vi "Configure Channel.vi"(8 "error in (no error)":errorcluster, 10 "DAQmx Task In":refnum<k21>, 11 "DAQmxThermocoupleChannel in":refnum<class "TCChannel.lvclass">) -> (0 "error out":errorcluster, 2 "DAQmx Task":refnum<k21>)   [LabVIEW 2020, in "VolatusDAQConfig.lvlib" / "TCChannel.lvclass"]
uses:
  TCChannel.lvclass
  VolatusConfig/VolatusConfigElement/VolatusConfigElement.lvclass
  VolatusConfig/Channel/Channel.lvclass
  <vilib>/DAQmx/create/channels.llb/DAQmx Create Channel (AI-Temperature-Thermocouple).vi
  C:/dev/lv20CE/relink/lv-volatus/VolatusDAQConfig/DAQmxChannel/DAQmxChannel.lvclass
  C:/dev/lv20CE/relink/lv-volatus/VolatusConfig/Channel/Channel.lvclass
  C:/dev/lv20CE/relink/lv-volatus/VolatusConfig/VolatusConfigElement/VolatusConfigElement.lvclass
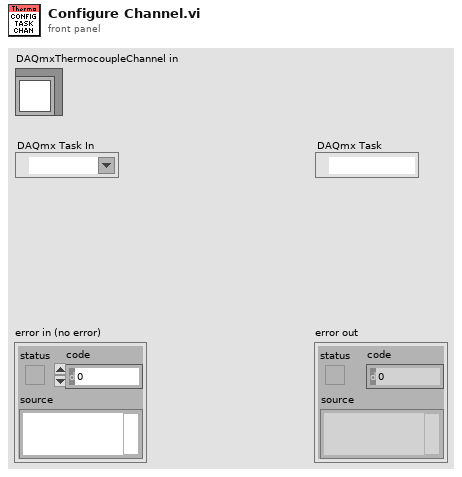
[diagram p1: front panel]
types:
  T1 = typedef "VolatusDAQConfig.lvlib/Temperature Units.ctl" = enum16{"C", "F", "K", "R"}
  T2 = typedef "VolatusDAQConfig.lvlib/TC Type.ctl" = enum16{"J", "K", "N", "R", "S", "T", "B", "E"}
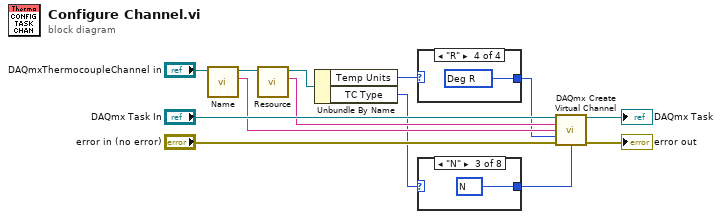
[diagram p0: block diagram]
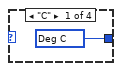
[diagram p2: hidden frame]
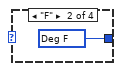
[diagram p3: hidden frame]
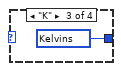
[diagram p4: hidden frame]
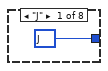
[diagram p5: hidden frame]
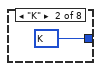
[diagram p6: hidden frame]
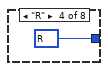
[diagram p7: hidden frame]
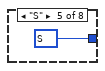
[diagram p8: hidden frame]
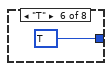
[diagram p9: hidden frame]
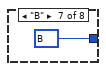
[diagram p10: hidden frame]
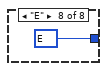
[diagram p11: hidden frame]
diagram:
  n1 = call "Name.vi"("VolatusConfigElement in"="DAQmxThermocoupleChannel in") -> ("Name"=w7:string, "VolatusConfigElement out"=w9:refnum<class "TCChannel.lvclass">)  [unwired: 8 in, 1 out]
  n2 = call "Resource.vi"("Channel in"=w9) -> ("Resource"=w6:string, "Channel out"=w5:refnum<class "TCChannel.lvclass">)  [unwired: 8 in, 1 out]
  n3 = Unbundle By Name(w5) -> ("Temp Units"=w2:T1, "TC Type"=w4:T2)
  n4 = case shown="\"R\"" w2 {
    tunnel: [w14 w15 w16 w17] -> w1
    frame "C" {
      w14 = 10143 items=["Deg C"=10143, "Deg F"=10144, "Kelvins"=10325, "Deg R"=10145, "From Custom Scale"=10065] ("units")
    }
    frame "F" {
      w15 = 10144 items=["Deg C"=10143, "Deg F"=10144, "Kelvins"=10325, "Deg R"=10145, "From Custom Scale"=10065] ("units")
    }
    frame "K" {
      w16 = 10325 items=["Deg C"=10143, "Deg F"=10144, "Kelvins"=10325, "Deg R"=10145, "From Custom Scale"=10065] ("units")
    }
    frame "R" {
      w17 = 10145 items=["Deg C"=10143, "Deg F"=10144, "Kelvins"=10325, "Deg R"=10145, "From Custom Scale"=10065] ("units")
    }
  }
  n5 = case shown="\"N\"" w4 {
    tunnel: [w18 w19 w20 w21 w22 w23 w24 w25] -> w3
    frame "J" {
      w18 = 10072 items=["J"=10072, "K"=10073, "N"=10077, "R"=10082, "S"=10085, "T"=10086, "B"=10047, "E"=10055] ("thermocouple type")
    }
    frame "K" {
      w19 = 10073 items=["J"=10072, "K"=10073, "N"=10077, "R"=10082, "S"=10085, "T"=10086, "B"=10047, "E"=10055] ("thermocouple type")
    }
    frame "N" {
      w20 = 10077 items=["J"=10072, "K"=10073, "N"=10077, "R"=10082, "S"=10085, "T"=10086, "B"=10047, "E"=10055] ("thermocouple type")
    }
    frame "R" {
      w21 = 10082 items=["J"=10072, "K"=10073, "N"=10077, "R"=10082, "S"=10085, "T"=10086, "B"=10047, "E"=10055] ("thermocouple type")
    }
    frame "S" {
      w22 = 10085 items=["J"=10072, "K"=10073, "N"=10077, "R"=10082, "S"=10085, "T"=10086, "B"=10047, "E"=10055] ("thermocouple type")
    }
    frame "T" {
      w23 = 10086 items=["J"=10072, "K"=10073, "N"=10077, "R"=10082, "S"=10085, "T"=10086, "B"=10047, "E"=10055] ("thermocouple type")
    }
    frame "B" {
      w24 = 10047 items=["J"=10072, "K"=10073, "N"=10077, "R"=10082, "S"=10085, "T"=10086, "B"=10047, "E"=10055] ("thermocouple type")
    }
    frame "E" {
      w25 = 10055 items=["J"=10072, "K"=10073, "N"=10077, "R"=10082, "S"=10085, "T"=10086, "B"=10047, "E"=10055] ("thermocouple type")
    }
  }
  n6 = call-poly <vilib>:"DAQmx Create Virtual Channel.vi"("task in"="DAQmx Task In", "physical channels"=w6, "name to assign"=w7, "units"=w1, "error in"="error in (no error)", "thermocouple type"=w3) -> ("task out"=→"DAQmx Task":refnum<k21>, "error out"=→"error out":errorcluster)  [unwired: 8 in]
